vi "Write.vi"(6 "error in":errorcluster, 7 "Messages":T2[](array[typedef]), 8 "Number to Write":i32, 9 "CanHandleIn":T1) -> (0 "error out":errorcluster, 3 "CanHandleOut":T1)   [LabVIEW 2011, in "Konvolucio MCAN120803.lvlib"]
doc: "Writes data from a frame buffer to the bus."
uses:
  <instrlib>/Konvolucio MCAN120803/Konvolucio MCAN120803.lvlib
  <instrlib>/Konvolucio MCAN120803/Types/MessageType.ctl
  <instrlib>/Konvolucio MCAN120803/Types/CanHandleType.ctl
  C:/Program Files/National Instruments/LabVIEW 2011/instr.lib/Konvolucio MCAN120803/Private/Konvolucio.MCAN120803.API.dll
  Private/Konvolucio.MCAN120803.API.dll
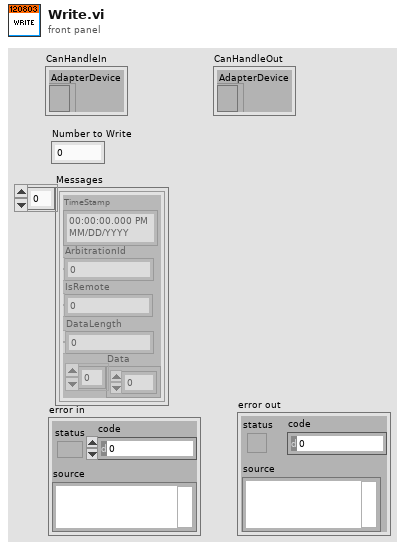
[diagram p1: front panel]
types:
  T1 = typedef "Konvolucio MCAN120803.lvlib/CanHandleType.ctl" = cluster{"AdapterDevice":refnum<k24>}
  T2 = typedef "Konvolucio MCAN120803.lvlib/MessageType.ctl" = cluster{"TimeStamp":timestamp, "ArbitrationId":u32, "IsRemote":u8, "DataLength":u8, "Data":u8[]}
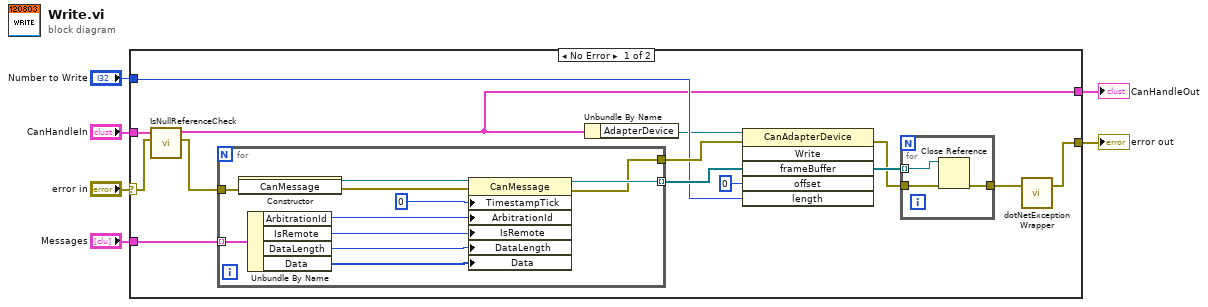
[diagram p0: block diagram]
diagram:
  n1 = case shown="No Error" "error in" {
    selector: "error in" -> [w9 w36]
    tunnel: [w13 w36] -> w6
    tunnel: "Messages" -> [w18 _]
    tunnel: "Number to Write" -> [w14 _]
    tunnel: [w7 w35] -> w2
    tunnel: "CanHandleIn" -> [w10 w35]
    frame No Error {
      n2 = call <instrlib>:"IsNullReferenceCheck.vi"("error in"=w9, "MCanHandleIn"=w10) -> ("error out"=w8:errorcluster, "MCanHandleOut"=w7:T1)  [unwired: 5 in]
      n3 = for {
        tunnel: [w24] -> w17
        tunnel: [w25] -> w19 mode=indexing
        tunnel: w8 -> [w34]
        tunnel: w18 -> [w33] mode=indexing
        n4 = constructor class="CanMessage"(error in=w34) -> (reference out=w32:refnum<k24>, error out=w31:errorcluster)  [unwired: 2 in, 1 out]
        n5 = Unbundle By Name(w33) -> ("ArbitrationId"=w29:u32, "IsRemote"=w28:u8, "DataLength"=w27:u8, "Data"=w26:u8[])
        n6 = property class="CanMessage"(reference=w32, error in=w31, "TimestampTick"=i64 0 ("Timestamp"), "ArbitrationId"=w29, "IsRemote"=w28, "DataLength"=w27, "Data"=w26) -> (reference out=w25:refnum<k24>, error out=w24:errorcluster)
      }
      n7 = Unbundle By Name(w7) -> ("AdapterDevice"=w11:refnum<k24>)
      n8 = invoke class="CanAdapterDevice" method="Write"(reference=w11, error in=w17, "frameBuffer"=w19, "offset"=0, "length"=w14) -> (error out=w15:errorcluster, "frameBuffer"=w16:refnum<k24>[])  [unwired: 1 in, 4 out]
      n9 = for {
        tunnel: w16 -> [w22] mode=indexing
        tunnel: w15 -> [w23]
        tunnel: [w21] -> w12
        n10 = Close Reference(reference=w22, error in (no error)=w23) -> (error out=w21:errorcluster)
      }
      n11 = call <instrlib>:"dotNetExceptionWrapper.vi"("error in"=w12) -> ("error out"=w13:errorcluster)  [unwired: 2 in]
    }
    frame Error {
    }
  }
  "error out" <- w6
  "CanHandleOut" <- w2
